vi "host.vi"() -> ()   [LabVIEW 2020]
uses:
  <vilib>/Utility/file.llb/Write Delimited Spreadsheet (DBL).vi
panel:
  in  "y predict save":path
  out "total time (s)":dbl
  out "max iteration":dbl
  out "iteration":dbl
  out "X":dbl[][](array[numeric])
  in  "X data filepath":path
  in  "stop":bool
  out "y waveform":cluster{"Numeric":dbl, "Double":dbl}(graph)
  out "y":dbl[][](array[numeric])
  in  "y data filepath":path
  out "Waveform Graph":dbl[][](graph)
  out "y predict values":dbl[](array[numeric])
  out "x waveform":dbl[](graph)
  out "t":dbl[][](array[numeric])
  in  "t data filepath":path
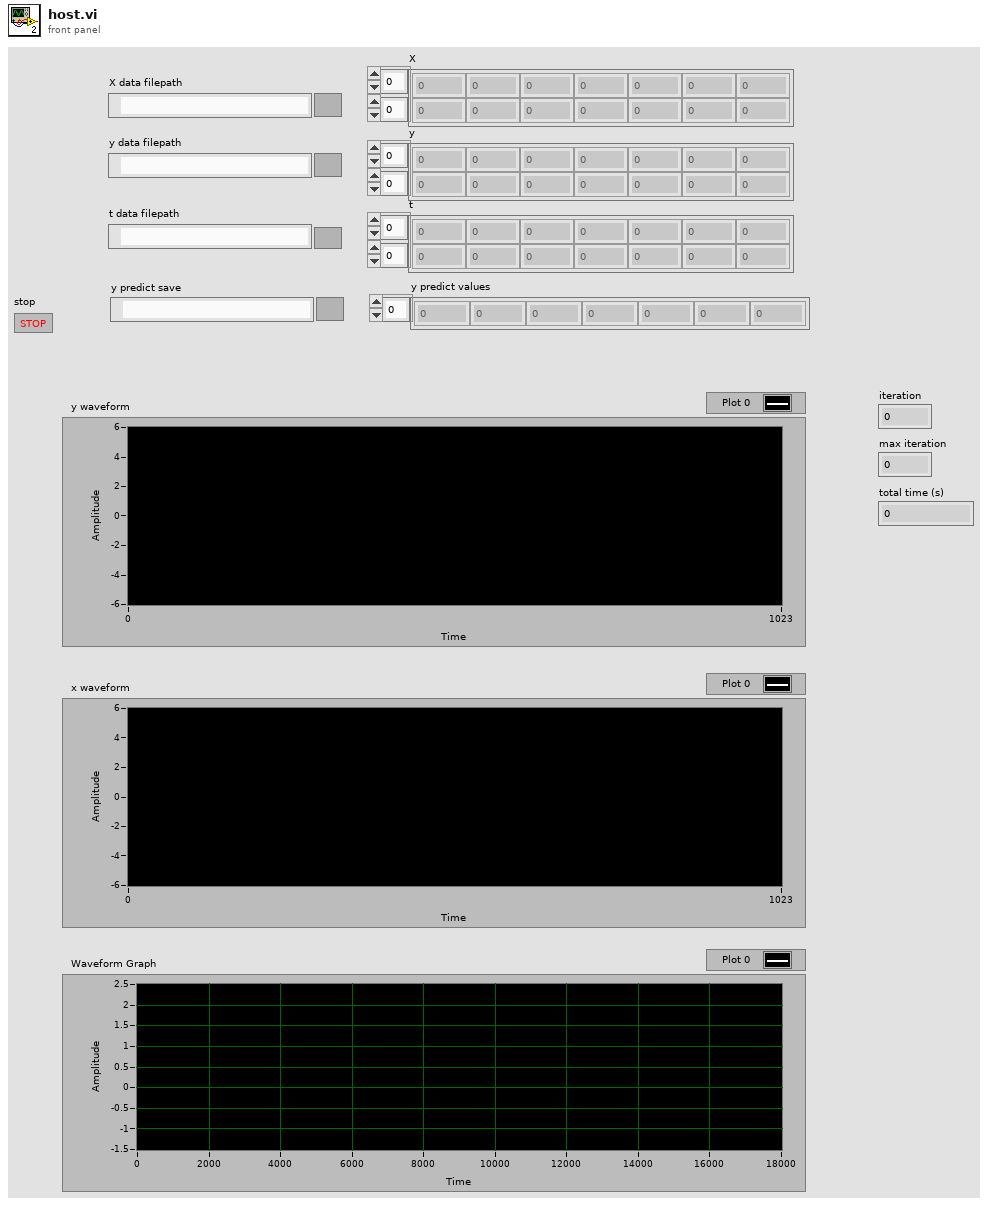
[diagram p1: front panel]
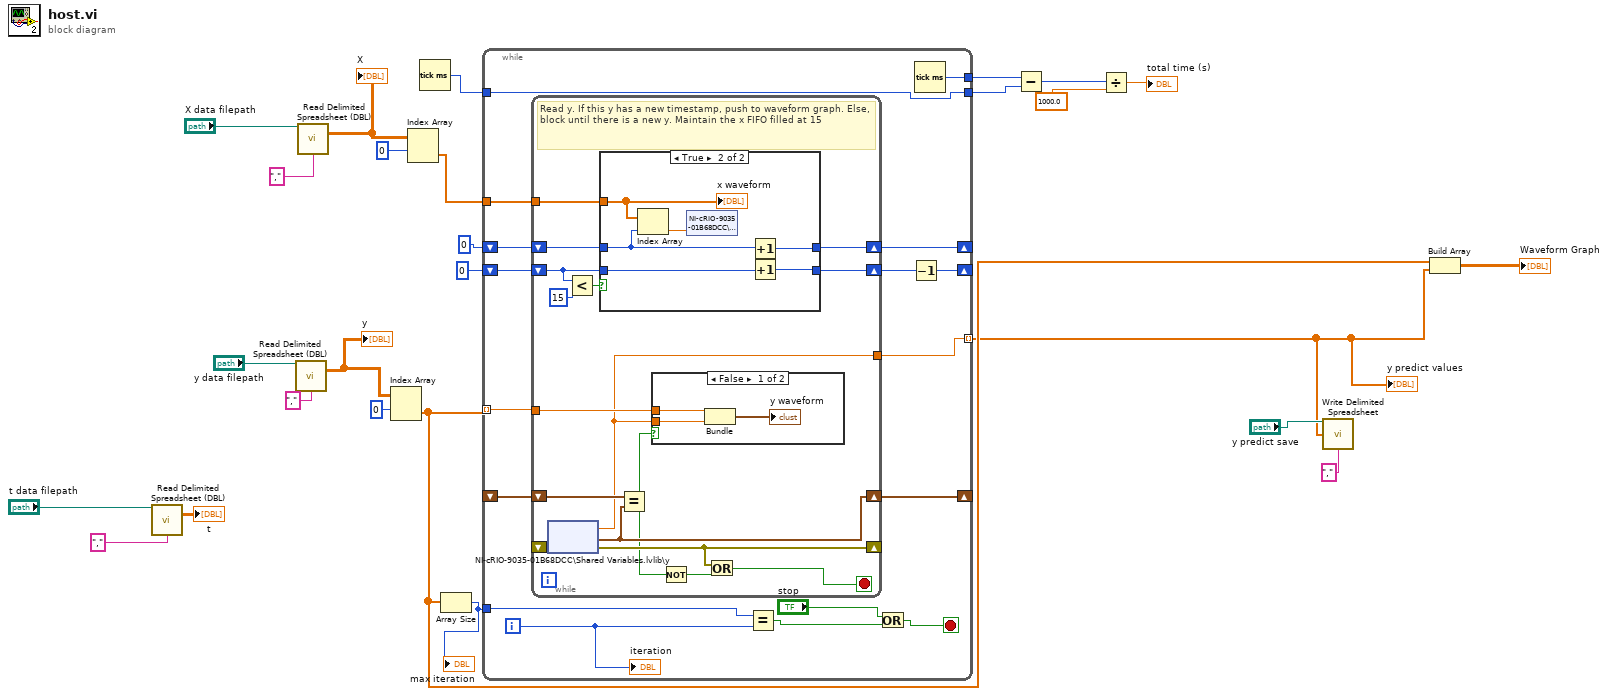
[diagram p0: block diagram]
diagram:
  n1 = call <vilib>:"Read Delimited Spreadsheet (DBL).vi"("file path (dialog if empty)"="t data filepath", "delimiter (\\t)"=",") -> ("all rows"=→"t":dbl[][])  [unwired: 8 in, 5 out]
  n2 = call <vilib>:"Read Delimited Spreadsheet (DBL).vi"("file path (dialog if empty)"="y data filepath", "delimiter (\\t)"=",") -> ("all rows"=w19:dbl[][])  [unwired: 8 in, 5 out]
  "y" <- w19
  n3 = call <vilib>:"Read Delimited Spreadsheet (DBL).vi"("file path (dialog if empty)"="X data filepath", "delimiter (\\t)"=",") -> ("all rows"=w16:dbl[][])  [unwired: 8 in, 5 out]
  "X" <- w16
  n4 = Index Array(array=w19, index (row)=0) -> (element=w14:dbl[])  [unwired: 1 in]
  n5 = Index Array(array=w16, index (row)=0) -> (element=w12:dbl[])  [unwired: 1 in]
  n6 = Tick Count (ms)() -> (millisecond timer value=w9:u32)
  n7 = Array Size(array=w14) -> (size(s)=w13:i32)
  "max iteration" <- w13
  n8 = while {
    tunnel: w14 -> [w43] mode=indexing
    tunnel: [w40] -> w2 mode=indexing
    shift-right: [w42] -> _
    shift-left: _ -> [w41]
    tunnel: w13 -> [w39]
    tunnel: w12 -> [w34]
    shift-right: [w32] -> _
    shift-left: 0 -> [w33]
    shift-right: [w30] -> _
    shift-left: 0 -> [w31]
    tunnel: w9 -> [w28]
    tunnel: [w28] -> w4
    tunnel: [w27] -> w5
    i -> [w35]
    stop <- w37 stop-if-true
    n9 = while {
      shift-right: [w58] -> w42
      shift-left: w41 -> [w57]
      shift-right: [w56] -> _
      shift-left: _ -> [w59]
      tunnel: w43 -> [w53]
      tunnel: [w52] -> w40
      tunnel: w34 -> [w50]
      shift-right: [w48] -> w32
      shift-left: w33 -> [w49]
      shift-right: [w47] -> w29
      shift-left: w31 -> [w45]
      stop <- w51 stop-if-true
      # "Read y. If this y has a new timestamp, push to waveform graph. Else, block until there is a new y. Maintain the x FIFO filled at 15"
      n10 = shared-variable "NI-cRIO-9035-01B68DCC\\Shared Variables.lvlib\\y"(error in=w59) -> (w52:dbl, error out=w56:errorcluster, w58:timestamp)
      n11 = Less?(x=w45, y=15) -> (x < y?=w44:bool)
      n12 = case shown="True" w44 {
        tunnel: w50 -> [_ w67]
        tunnel: w49 -> [w61 w65]
        tunnel: [w61 w64] -> w48
        tunnel: w45 -> [w60 w63]
        tunnel: [w60 w62] -> w47
        frame False {
        }
        frame True {
          n13 = Index Array(array=w67, index=w65) -> (element=w66:dbl)
          n14 = shared-variable "NI-cRIO-9035-01B68DCC\\Shared Variables.lvlib\\x"(w66) -> ()  [unwired: 1 in, 1 out]
          n15 = Increment(x=w65) -> (x+1=w64:i32)
          n16 = Increment(x=w63) -> (x+1=w62:i32)
          "x waveform" <- w67
        }
      }
      n17 = Equal?(x=w57, y=w58) -> (x = y?=w54:bool)
      n18 = case shown="False" w54 {
        tunnel: w53 -> [w69 _]
        tunnel: w52 -> [w68 _]
        frame False {
          n19 = Bundle("Numeric"=w69, "Double"=w68) -> (→"y waveform":cluster{"Numeric":dbl, "Double":dbl})  [unwired: 1 in]
        }
        frame True {
        }
      }
      n20 = Not(x=w54) -> (.not. x?=w55:bool)
      n21 = Or(x=w56, y=w55) -> (x .or. y?=w51:bool)
    }
    n22 = Equal?(x=w39, y=w35) -> (x = y?=w36:bool)
    n23 = Or(x="stop", y=w36) -> (x .or. y?=w37:bool)
    n24 = Decrement(x=w29) -> (x-1=w30:i32)
    n25 = Tick Count (ms)() -> (millisecond timer value=w27:u32)
    "iteration" <- w35
  }
  "y predict values" <- w2
  n26 = Subtract(x=w5, y=w4) -> (x-y=w8:u32)
  n27 = Divide(x=w8, y=1000.0) -> (x/y=→"total time (s)":dbl)
  n28 = call-poly <vilib>:"Write Delimited Spreadsheet.vi"("file path (dialog if empty)"="y predict save", "1D data"=w2, "delimiter (\\t)"=",") -> ()  [unwired: 11 in, 2 out]
  n29 = Build Array(w14, w2) -> (→"Waveform Graph":dbl[][])
